vi "Write log thresholds.vi"(8 "error in (no error)":errorcluster, 10 "log thresholds":T1, 11 "Log Producer in":refnum<class "Log Producer.lvclass">) -> (0 "error out":errorcluster, 3 "Log Producer out":refnum<class "Log Producer.lvclass">)   [LabVIEW 2020, in "AIM ARINC 664 Engine.lvlib" / "Implementation.lvlib" / "Frame Logging.lvlib" / "Log Producer.lvclass"]
uses:
  Log Producer.lvclass
  Log Producer.lvclass/Log Producer.ctl
  Shared/FileSegmentType.ctl
  Monitor Execution Unit/loggingThreshold_types.ctl
  Monitor Execution Unit/Monitor Execution Unit.lvclass
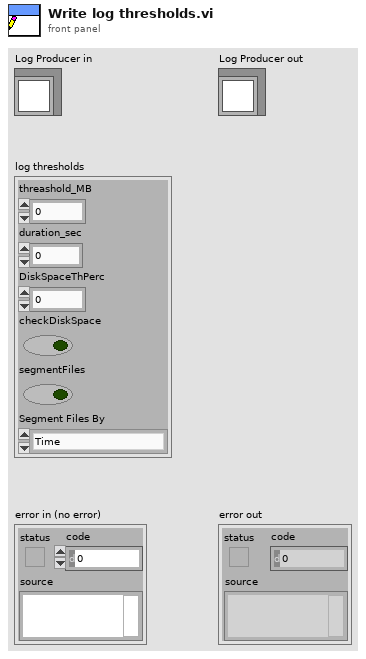
[diagram p1: front panel]
types:
  T1 = typedef "AIM ARINC 664 Engine.lvlib/Implementation.lvlib/Monitor Execution Unit.lvclass/loggingThreshold_types.ctl" = cluster{"threashold_MB":dbl, "duration_sec":dbl, "DiskSpaceThPerc":dbl, "checkDiskSpace":bool, "segmentFiles":bool, "Segment Files By":T2}
  T2 = typedef "FileSegmentType.ctl" = enum16{"Time", "Size"}
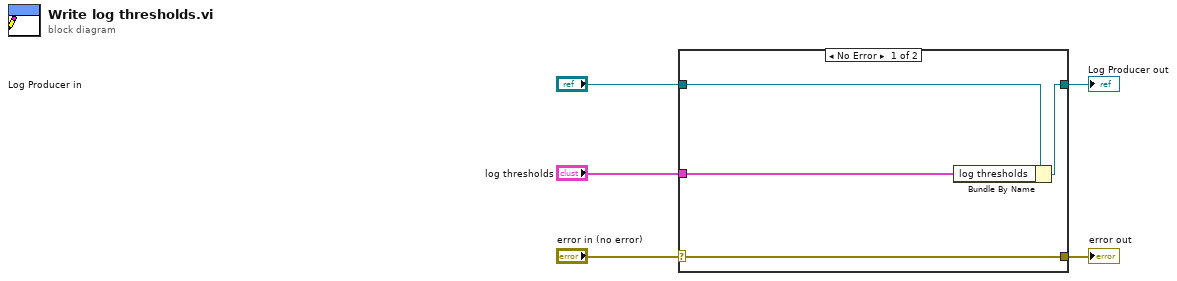
[diagram p0: block diagram]
diagram:
  n1 = case shown="No Error" "error in (no error)" {
    selector: "error in (no error)" -> [w9 w10]
    tunnel: [w9 w10] -> w4
    tunnel: [w7 w11] -> w2
    tunnel: "Log Producer in" -> [w8 w11]
    tunnel: "log thresholds" -> [w6 _]
    frame No Error {
      n2 = Bundle By Name(cluster=w8, "log thresholds"=w6) -> (w7:refnum<class "Log Producer.lvclass">)
    }
    frame Error {
    }
  }
  "error out" <- w4
  "Log Producer out" <- w2
